vi "MultiDiagramTunnels.vi"(10 "Terminal Map In":map{string, T3}(c390), 11 "cluster in":T1) -> (2 "Terminal Map Out":map{string, T3}(c390), 3 "cluster out":T1)   [LabVIEW 2025]
uses:
  bd.ctl
  Node/Node.lvclass
  wire.ctl
  Terminal.ctl
  MultiDiagramStructure/MultiDiagramStructure.lvclass
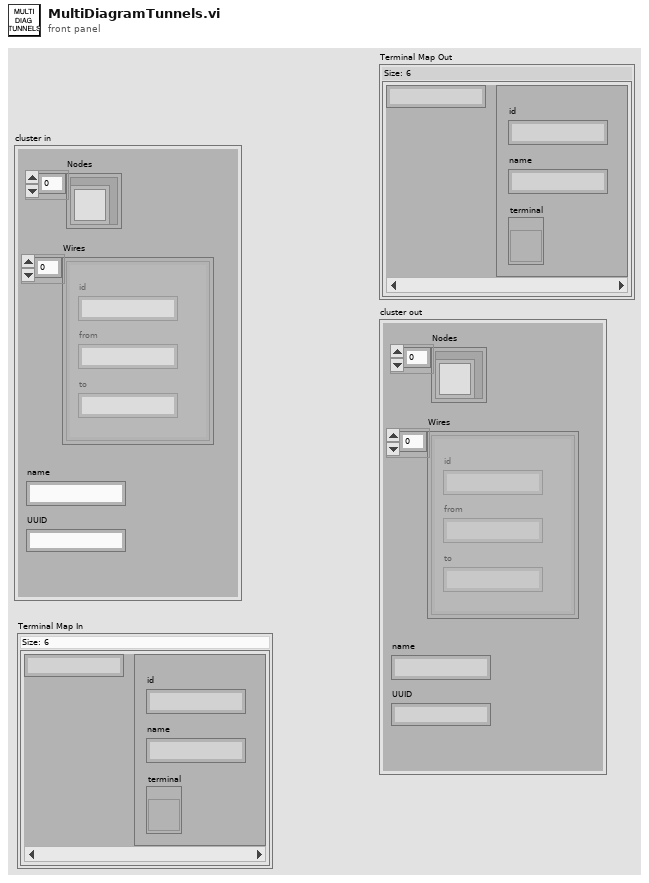
[diagram p1: front panel]
types:
  T1 = typedef "bd.ctl" = cluster{"Nodes":refnum<class "Node.lvclass">[], "Wires":T2[], "name":string, "UUID":string}
  T2 = typedef "wire.ctl" = cluster{"id":string, "from":string, "to":string}
  T3 = typedef "Terminal.ctl" = cluster{"id":string, "name":string, "terminal":refnum<vi>}
  T4 = typedef "Tunnel.ctl" = cluster{"OuterUUID":string, "InnerUUIDs":string[]}
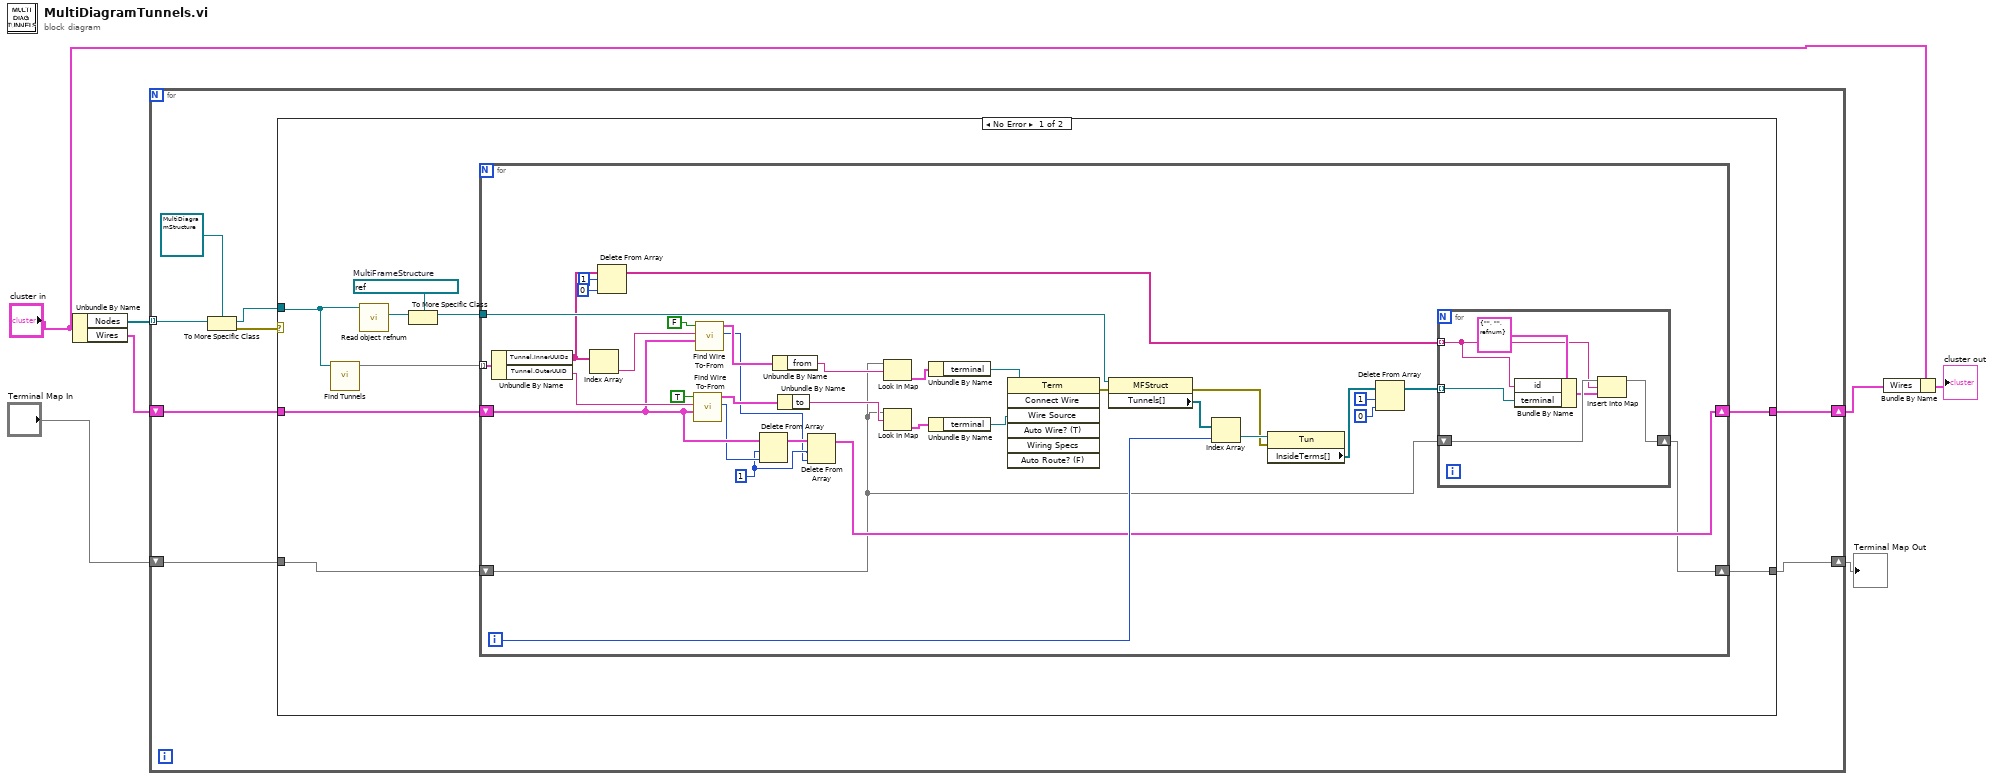
[diagram p0: block diagram]
diagram:
  n1 = Unbundle By Name("cluster in") -> ("Nodes"=w7:refnum<class "Node.lvclass">[], "Wires"=w5:T2[])
  n2 = for {
    tunnel: w7 -> [w15] mode=indexing
    shift-right: [w8] -> w4
    shift-left: "Terminal Map In" -> [w11]
    shift-right: [w9] -> w1
    shift-left: w5 -> [w10]
    n3 = To More Specific Class(target class=refnum<class "MultiDiagramStructure.lvclass"> refnum ("MultiDiagramStructure.lvclass"), reference=w15) -> (specific class reference=w12:refnum<class "MultiDiagramStructure.lvclass">, error out=w13:errorcluster)  [unwired: 1 in]
    n4 = case shown="No Error" w13 {
      tunnel: w12 -> [w24 _]
      tunnel: w11 -> [w21 w66]
      tunnel: w10 -> [w19 w67]
      tunnel: [w17 w67] -> w9
      tunnel: [w16 w66] -> w8
      frame No Error {
        w22 = refnum<vi> refnum  # MultiFrameStructure
        n5 = call "Find Tunnels.vi"("MultiDiagramStructure in"=w24) -> ("Tunnels"=w20:map{string, T4})  [unwired: 10 in]
        n6 = call-dynamic "Read object refnum.vi"("Node in"=w24) -> ("object refnum"=w23:refnum<vi>)  [unwired: 8 in, 2 out]
        n7 = To More Specific Class(target class=w22, reference=w23) -> (specific class reference=w18:refnum<vi>)  [unwired: 1 in, 1 out]
        n8 = for {
          shift-right: [w25] -> w16
          shift-left: w21 -> [w26]
          tunnel: w20 -> [w59] mode=indexing
          tunnel: w18 -> [w46]
          shift-right: [w36] -> w17
          shift-left: w19 -> [w41]
          i -> [w44]
          w38 = 1 ("length")
          n9 = Unbundle By Name(w59) -> ("Tunnel.InnerUUIDs"=w34:string[], "Tunnel.OuterUUID"=w58:string)
          n10 = Index Array(array=w34) -> (element=w35:string)  [unwired: 1 in]
          n11 = Delete From Array(array=w34, length=1, index=0) -> (array with subset deleted=w28:string[])  [unwired: 1 out]
          n12 = call "Find Wire To-From.vi"("Wires"=w41, "termUUID"=w58, "From UUID?"=TRUE) -> ("Index"=w40:i32, "Wire"=w54:T2)  [unwired: 7 in]
          n13 = call "Find Wire To-From.vi"("Wires"=w41, "termUUID"=w35, "From UUID?"=FALSE) -> ("Index"=w37:i32, "Wire"=w55:T2)  [unwired: 7 in]
          n14 = Delete From Array(array=w41, length=w38, index=w40) -> (array with subset deleted=w39:T2[])  [unwired: 1 out]
          n15 = Unbundle By Name(w55) -> ("from"=w53:string)
          n16 = Unbundle By Name(w54) -> ("to"=w52:string)
          n17 = Delete From Array(array=w39, length=w38, index=w37) -> (array with subset deleted=w36:T2[])  [unwired: 1 out]
          n18 = Look In Map(map=w26, key=w53) -> (value=w50:T3)  [unwired: 1 in, 1 out]
          n19 = Look In Map(map=w26, key=w52) -> (value=w51:T3)  [unwired: 1 in, 1 out]
          n20 = Unbundle By Name(w50) -> ("terminal"=w49:refnum<vi>)
          n21 = Unbundle By Name(w51) -> ("terminal"=w48:refnum<vi>)
          n22 = invoke class="Term" method="Connect Wire"(reference=w49, "Wire Source"=w48) -> (error out=w47:errorcluster)  [unwired: 5 in, 6 out]
          n23 = property class="MFStruct"(reference=w46, error in=w47) -> (error out=w42:errorcluster, "Tunnels[]"=w45:refnum<vi>[])  [unwired: 1 out]
          n24 = Index Array(array=w45, index=w44) -> (element=w43:refnum<vi>)
          n25 = property class="Tun"(reference=w43, error in=w42) -> ("InsideTerms[]"=w31:refnum<vi>[])  [unwired: 2 out]
          n26 = Delete From Array(array=w31, length=1, index=0) -> (array with subset deleted=w27:refnum<vi>[])  [unwired: 1 out]
          n27 = for {
            tunnel: w28 -> [w62] mode=indexing
            tunnel: w27 -> [w63] mode=indexing
            shift-right: [w61] -> w25
            shift-left: w26 -> [w65]
            n28 = Bundle By Name(cluster=T3 {"id"="", "name"="", "terminal"=refnum} ("value"), "id"=w62, "terminal"=w63) -> (w60:T3)
            n29 = Insert Into Map(map in=w65, key=w62, value=w60) -> (map out=w61:map{string, T3})  [unwired: 2 out]
          }
        }
      }
      frame Error {
      }
    }
  }
  "Terminal Map Out" <- w4
  n30 = Bundle By Name(cluster="cluster in", "Wires"=w1) -> (→"cluster out":T1)
